vi "ISEG_HVSystemGUI.contents.vi"   [LabVIEW 2014, in "ISEG_HVSystemGUI.lvlib"]
doc: "loads all VIs of a class into memory - required for building applications"
uses:
  ISEG_HVSystemGUI.lvlib
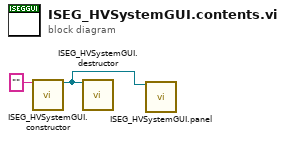
[diagram p0: block diagram]
diagram:
  n1 = call "ISEG_HVSystemGUI.constructor.vi"("name"="") -> ("i ref out"=w1:refnum<vi>)  [unwired: 16 in, 2 out]
  n2 = call "ISEG_HVSystemGUI.destructor.vi"("i ref in"=w1) -> ()  [unwired: 18 in, 1 out]
  n3 = call "ISEG_HVSystemGUI.panel.vi"("object ref"=w1) -> ()  [unwired: 18 in, 1 out]
